vi "pdf_function_m.vi"(3 "u":dbl format="%.2f", 4 "v":dbl format="%.2f", 5 "w":dbl format="%.2f", 8 "Initialise":bool) -> (14 "F":dbl format="%.5f")   [LabVIEW 2010]
uses:
  xw_correction_global_m.vi
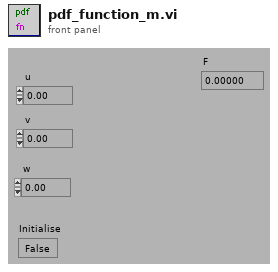
[diagram p1: front panel]
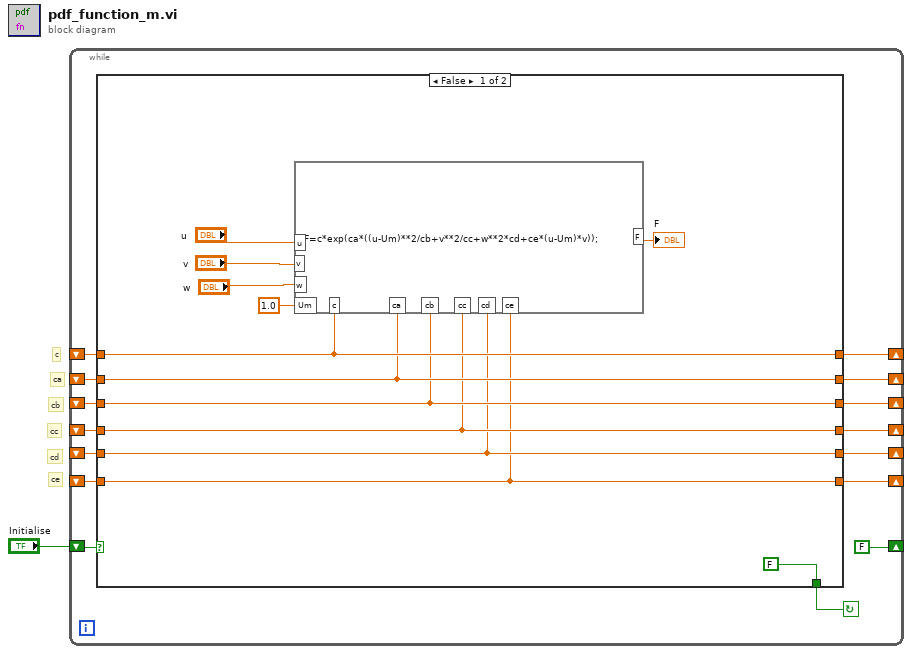
[diagram p0: block diagram]
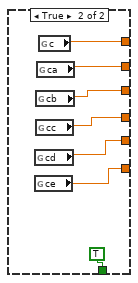
[diagram p2: hidden frame]
diagram:
  # "c"
  # "ce"
  # "cd"
  # "cc"
  # "cb"
  # "ca"
  n1 = while {
    shift-left: _ -> [w6]
    shift-right: [w5] -> _
    shift-left: _ -> [w7]
    shift-right: [w4] -> _
    shift-left: _ -> [w8]
    shift-right: [w3] -> _
    shift-left: _ -> [w9]
    shift-right: [w2] -> _
    shift-left: _ -> [w11]
    shift-right: [w10] -> _
    shift-left: _ -> [w13]
    shift-right: [w12] -> _
    shift-left: "Initialise" -> [w16]
    shift-right: [FALSE] -> _
    stop <- w15 continue-if-true
    n2 = case shown="False" w16 {
      tunnel: [FALSE TRUE] -> w15
      tunnel: w13 -> [w22 _]
      tunnel: [w22 w29] -> w12
      tunnel: w11 -> [w21 _]
      tunnel: [w21 w30] -> w10
      tunnel: w9 -> [w20 _]
      tunnel: w8 -> [w19 _]
      tunnel: w7 -> [w18 _]
      tunnel: w6 -> [w17 _]
      tunnel: [w17 w34] -> w5
      tunnel: [w18 w33] -> w4
      tunnel: [w19 w32] -> w3
      tunnel: [w20 w31] -> w2
      frame False {
        n3 = formula code="F=c*exp(ca*((u-Um)**2/cb+v**2/cc+w**2*cd+ce*(u-Um)*v));"("c"=w22, "u"="u", "v"="v", "w"="w", "Um"=1.0, "ca"=w21, "cb"=w20, "cc"=w19, "cd"=w18, "ce"=w17) -> ("F"=→"F":dbl)
      }
      frame True {
        n4 = global read "xw_correction_global_m.vi" "cd"() -> (w33:dbl)
        n5 = global read "xw_correction_global_m.vi" "ce"() -> (w34:dbl)
        n6 = global read "xw_correction_global_m.vi" "cb"() -> (w31:dbl)
        n7 = global read "xw_correction_global_m.vi" "cc"() -> (w32:dbl)
        n8 = global read "xw_correction_global_m.vi" "ca"() -> (w30:dbl)
        n9 = global read "xw_correction_global_m.vi" "c"() -> (w29:dbl)
      }
    }
  }
